vi "Get Class C Description.vi"(8 "error in (no error)":errorcluster, 11 "LabVIEW Obj":refnum<class>) -> (0 "error out":errorcluster, 3 "resulting string":string)   [LabVIEW 2017]
uses:
  <userlib>/_OpenG.lib/string/string.llb/Multi-line String to Array__ogtk.vi
  String/LinesToText.vi
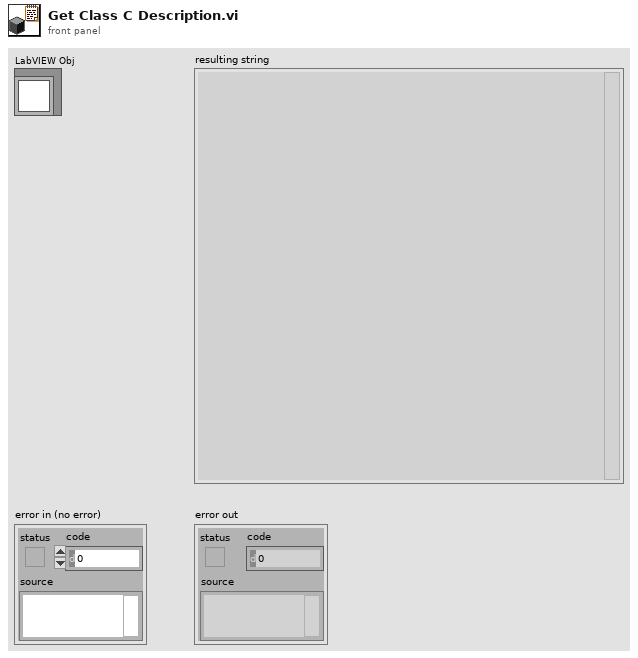
[diagram p1: front panel]
types:
  T1 = enum32{"invalid scope", "public", "private", "protected", "community"}[]
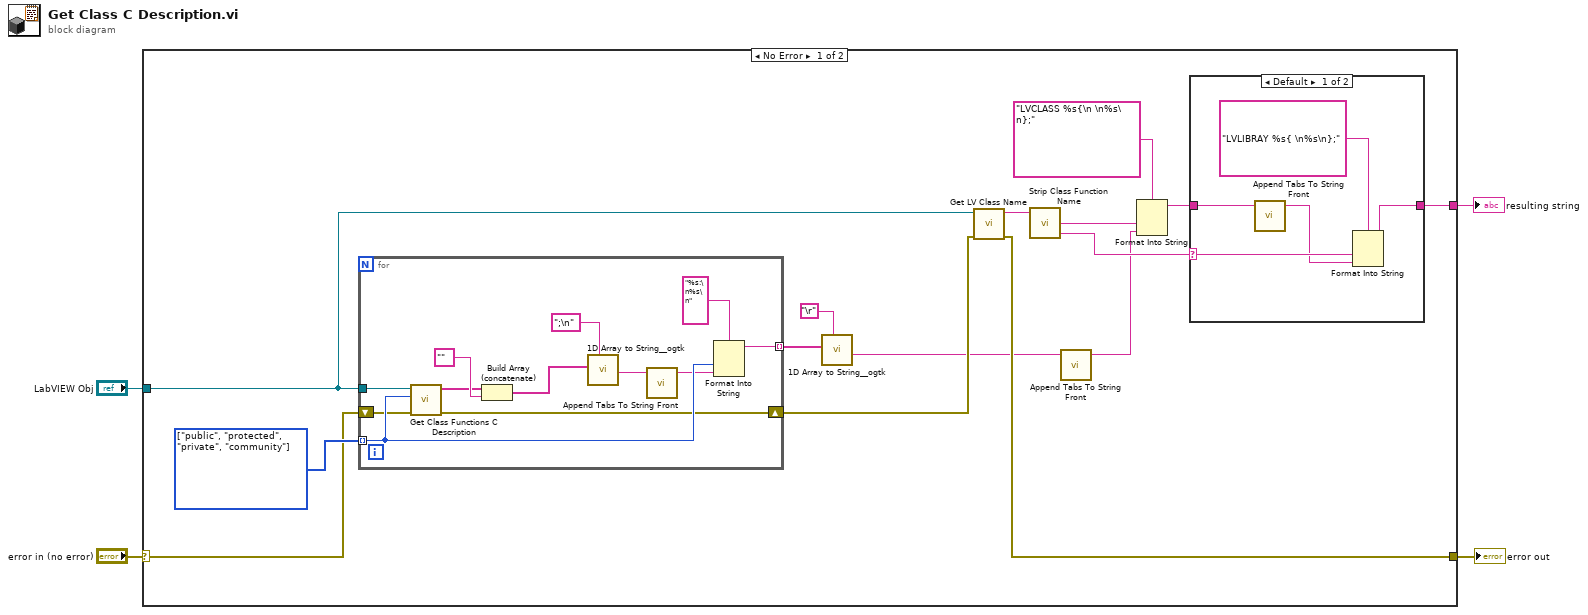
[diagram p0: block diagram]
diagram:
  n1 = case shown="No Error" "error in (no error)" {
    selector: "error in (no error)" -> [w13 w38]
    tunnel: "LabVIEW Obj" -> [w16 _]
    tunnel: [w8 _] -> w3
    tunnel: [w14 w38] -> w2
    frame No Error {
      w19 = T1 [enum."public", enum."protected", enum."private", enum."community"] items=["invalid scope", "public", "private", "protected", "community"] ("Access Scope")
      n2 = for {
        tunnel: w19 -> [w34] mode=indexing
        tunnel: [w33] -> w15 mode=indexing
        tunnel: w16 -> [w32]
        shift-right: [w29] -> w12
        shift-left: w13 -> [w30]
        n3 = call "Get Class Functions C Description.vi"("error in (no error)"=w30, "Access Scope"=w34, "LabVIEW Obj"=w32) -> ("error out"=w29:errorcluster, "Array"=w28:string[])  [unwired: 7 in]
        n4 = Build Array (concatenate)(w28, "" ("delimiter (Tab)")) -> (w36:string[])
        n5 = call <userlib>:"1D Array to String__ogtk.vi"("delimiter (Tab)"=";\n", "Array of Strings"=w36) -> ("delimited string"=w27:string)  [unwired: 9 in]
        n6 = call "Append Tabs To String Front.vi"("Str in"=w27) -> ("Str out"=w26:string)  [unwired: 4 in]
        n7 = Format Into String(format string="%s:\n%s\n", w34, w26) -> (resulting string=w33:string)  [unwired: 2 in, 1 out]
      }
      n8 = call <userlib>:"1D Array to String__ogtk.vi"("delimiter (Tab)"="\r" ("Carriage Return Constant"), "Array of Strings"=w15) -> ("delimited string"=w6:string)  [unwired: 9 in]
      n9 = call <vilib>:"Get LV Class Name.vi"("error in (no error)"=w12, "object"=w16) -> ("error out"=w14:errorcluster, "class name"=w11:string)  [unwired: 8 in]
      n10 = call "Strip Class Function Name.vi"("File Full Path Name"=w11) -> ("library name"=w9:string, "Class name"=w10:string)  [unwired: 2 in, 1 out]
      n11 = call "Append Tabs To String Front.vi"("Str in"=w6) -> ("Str out"=w5:string)  [unwired: 4 in]
      n12 = Format Into String(format string="LVCLASS %s{\n \n%s\n};" ("delimiter (Tab)"), w10, w5) -> (resulting string=w7:string)  [unwired: 2 in, 1 out]
      n13 = case shown="Default" w9 {
        selector: w9 -> [w22 _]
        tunnel: [w23 w25] -> w8
        tunnel: w7 -> [w21 w25]
        frame Default {
          n14 = call "Append Tabs To String Front.vi"("Str in"=w21) -> ("Str out"=w20:string)  [unwired: 4 in]
          n15 = Format Into String(format string="LVLIBRAY %s{ \n%s\n};" ("delimiter (Tab)"), w22, w20) -> (resulting string=w23:string)  [unwired: 2 in, 1 out]
        }
        frame "" {
        }
      }
    }
    frame Error {
    }
  }
  "resulting string" <- w3
  "error out" <- w2
